vi "Write Components Notifier.vi"(8 "error in (no error)":errorcluster, 10 "Components":refnum<class "Component.lvclass">[](array[class]), 11 "Item Ref in":T1 format="%.0x") -> (0 "error out":errorcluster, 3 "Item Ref out":T1 format="%.0x")   [LabVIEW 2017, in "DSF System Explorer.lvlib"]
uses:
  DSF System Explorer.lvlib
  <vilib>/NI Veristand/Custom Device API/Custom Device Item Ref.ctl
  DSF Core.lvlibp/Classes/Component/Component.lvclass
  <vilib>/NI Veristand/Custom Device API/Custom Device API.lvlib
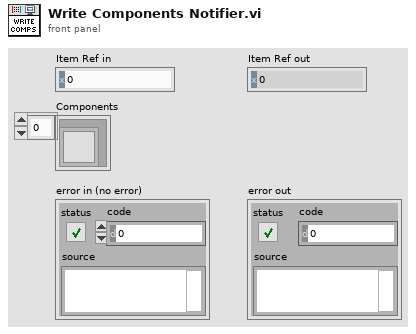
[diagram p1: front panel]
types:
  T1 = typedef "Custom Device API.lvlib/Custom Device Item Ref.ctl" = u64
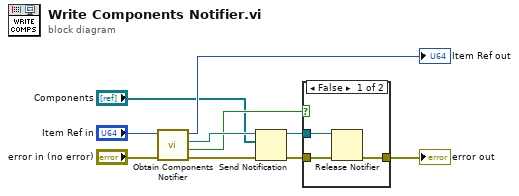
[diagram p0: block diagram]
diagram:
  n1 = call "Obtain Components Notifier.vi"("error in (no error)"="error in (no error)", "Item Ref in"="Item Ref in") -> ("error out"=w4:errorcluster, "created new?"=w2:bool, "comps notifier"=w3:refnum<notifier>, "Item Ref out"=→"Item Ref out":T1)  [unwired: 6 in]
  n2 = Send Notification(notification="Components", notifier=w3, error in (no error)=w4) -> (notifier out=w9:refnum<notifier>, error out=w10:errorcluster)
  n3 = case shown="False" w2 {
    tunnel: w10 -> [w13 w14]
    tunnel: w9 -> [w12 _]
    tunnel: [w11 w14] -> w8
    frame False {
      n4 = Release Notifier(notifier=w12, error in (no error)=w13) -> (error out=w11:errorcluster)  [unwired: 1 in, 2 out]
    }
    frame True {
    }
  }
  "error out" <- w8
